vi "WhetherValidMetrics.vi"(9 "Opstate":string, 10 "current metric":string) -> (2 "In valid list?":bool)   [LabVIEW 2017, in "McsaAnalysisLowRate.lvlib"]
uses:
  <vilib>/addons/InsightCM/Devices/Shared/Mcsa/McsaAnalysisLowRate/McsaAnalysisLowRate.lvlib
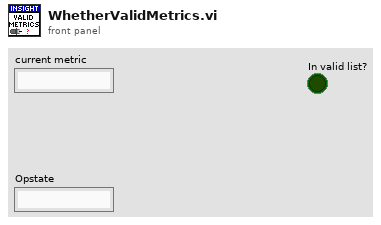
[diagram p1: front panel]
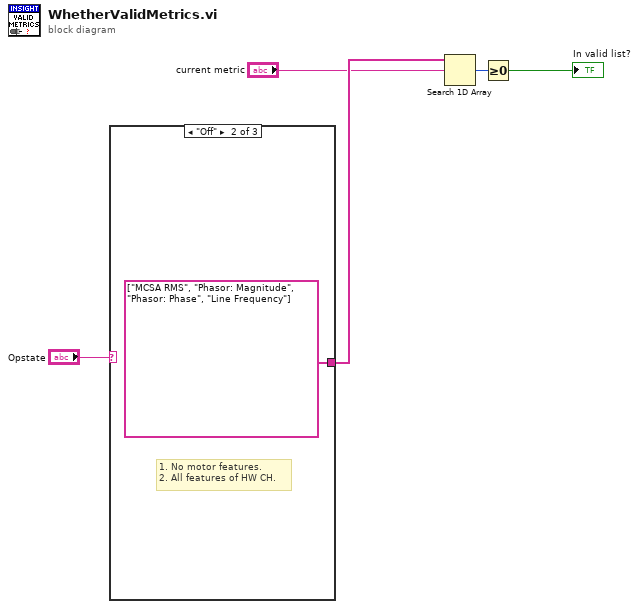
[diagram p0: block diagram]
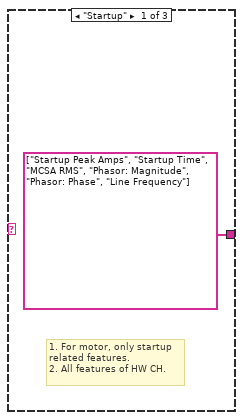
[diagram p2: hidden frame]
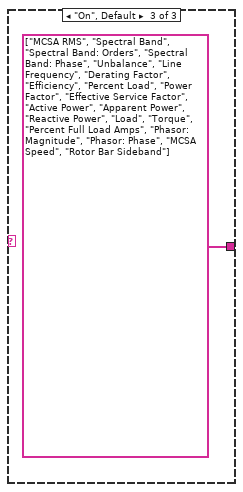
[diagram p3: hidden frame]
diagram:
  n1 = case shown="\"Off\"" "Opstate" {
    tunnel: [string[] ["Startup Peak Amps", "Startup Time", "MCSA RMS", "Phasor: Magnitude", "Phasor: Phase", "Line Frequency"] ("value") string[] ["MCSA RMS", "Phasor: Magnitude", "Phasor: Phase", "Line Frequency"] ("value") string[] ["MCSA RMS", "Spectral Band", "Spectral Band: Orders", "Spectral Band: Phase", "Unbalance", "Line Frequency", "Derating Factor", "Efficiency", "Percent Load", "Power Factor", "Effective Service Factor", "Active Power", "Apparent Power", "Reactive Power", "Load", "Torque", "Percent Full Load Amps", "Phasor: Magnitude", "Phasor: Phase", "MCSA Speed", "Rotor Bar Sideband"] ("value")] -> w5
    frame "Startup" {
      # "1. For motor, only startup\nrelated features.\n2. All features of HW CH."
    }
    frame "Off" {
      # "1. No motor features. \n2. All features of HW CH."
    }
    frame "On", Default {
    }
  }
  n2 = Search 1D Array(1D array=w5, element="current metric") -> (index of element=w4:i32)  [unwired: 1 in]
  n3 = Greater Or Equal To 0?(x=w4) -> (x >= 0?=→"In valid list?":bool)
